vi "_USB_CAN_DISP_ID_HB_.vi"(1 "arr new":T1[](array[typedef]), 2 "Reset buffer":bool, 3 "arr old":T1[](array[typedef])) -> (0 "Arr Out":T1[](array[typedef]))   [LabVIEW 2011]
uses:
  _USB_CAN_T_R_Unit_.ctl
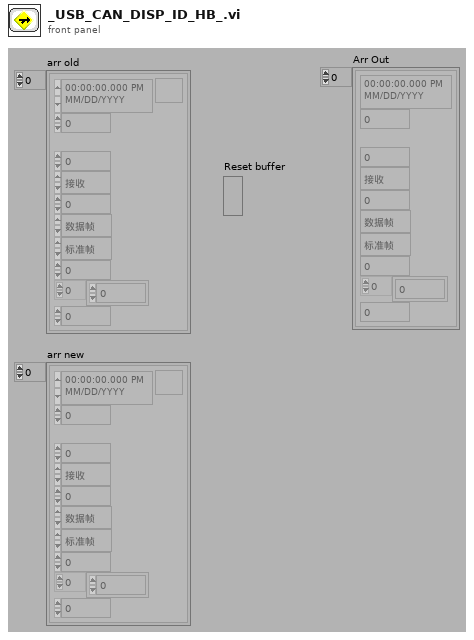
[diagram p1: front panel]
types:
  T1 = typedef "_USB_CAN_T_R_Unit_.ctl" = cluster{"time":timestamp, "channel":u16, "TimeStamp":u32, "tr":enum16{"接收", "发送"}, "id":u32, "Type":enum16{"数据帧", "远程帧"}, "Format":enum16{"标准帧", "扩展帧"}, "len":u8, "data":u8[], "sysTime":u32}
  T2 = cluster{"sysTime":u32, "channel":u16, "tr":enum16{"接收", "发送"}, "TR_Unit":T1}
  T3 = cluster{"sysTime":u32, "channel":u16, "tr":enum16{"接收", "发送"}, "TR_Unit":T1}[]
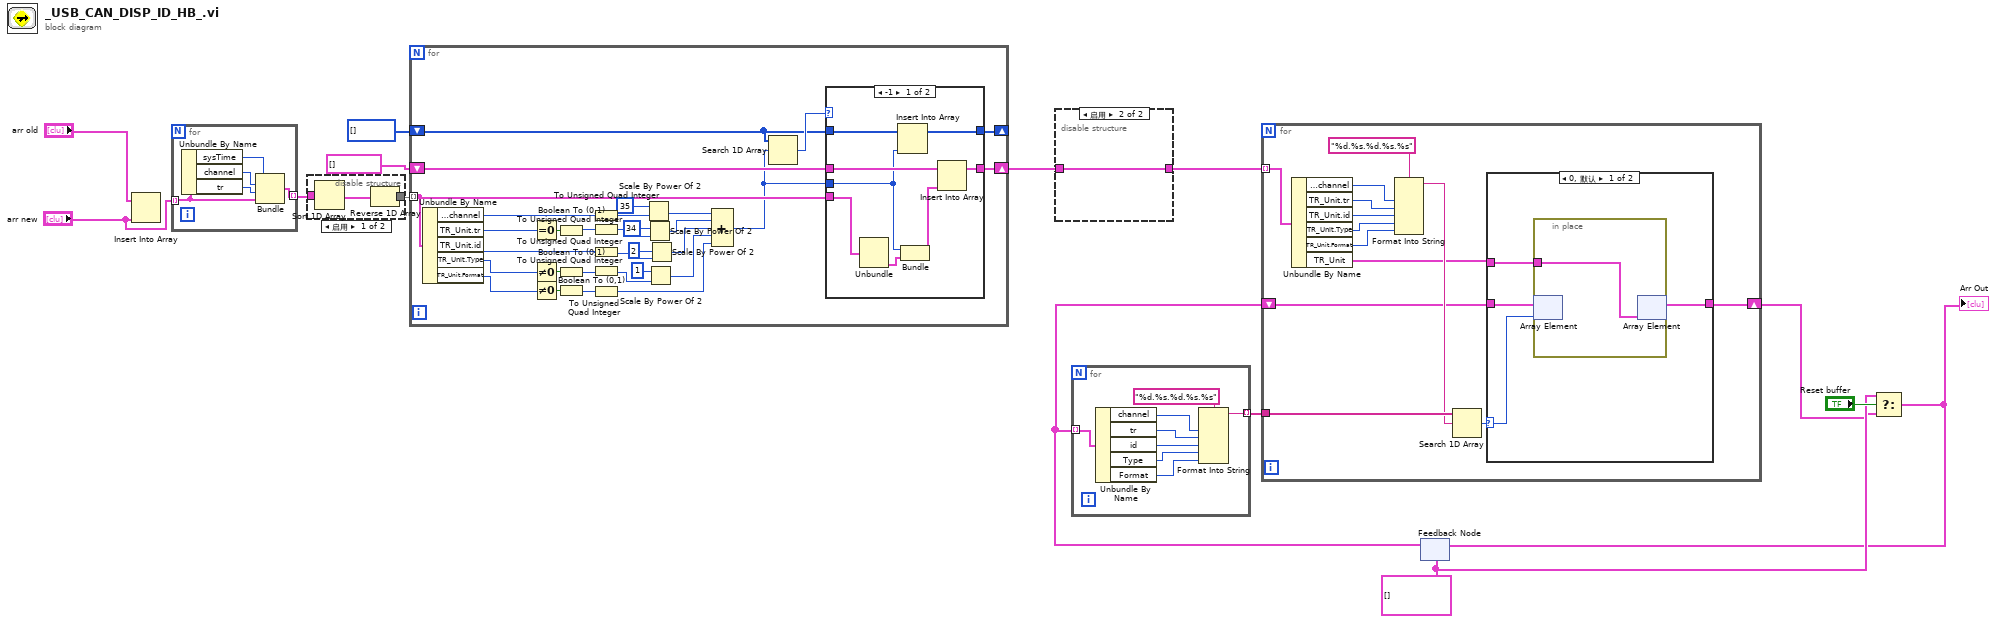
[diagram p0: block diagram]
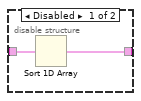
[diagram p2: hidden frame]
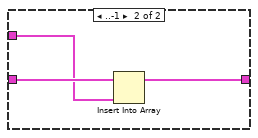
[diagram p4: hidden frame]
diagram:
  w4 = T1[] []
  n1 = Insert Into Array(array="arr old", new element="arr new") -> ()  [unwired: 1 in, 1 out]
  n2 = for {
    tunnel: "arr new" -> [w19] mode=indexing
    tunnel: [w17] -> w9 mode=indexing
    n3 = Unbundle By Name(w19) -> ("sysTime"=w15:u32, "channel"=w16:u16, "tr"=w18:enum16{"接收", "发送"})
    n4 = Bundle("sysTime"=w15, "channel"=w16, "tr"=w18, "TR_Unit"=w19) -> (w17:T2)  [unwired: 1 in]
  }
  n5 = disable-structure shown="启用" {
    disable-tunnel: w9 -> [w22 w23]
    disable-tunnel: [w20 w23] -> w8
    frame Enabled {
      n6 = Sort 1D Array(array=w22) -> (sorted array=w21:T3)
      n7 = Reverse 1D Array(array=w21) -> (reversed array=w20:T3)
    }
    frame Disabled {
    }
  }
  n8 = for {
    tunnel: w8 -> [w49] mode=indexing
    shift-right: [w52] -> w13
    shift-left: cluster{u64, "TR_Unit":T1}[] [] -> [w53]
    shift-right: [w50] -> _
    shift-left: u64[] [] -> [w51]
    n9 = Unbundle By Name(w49) -> ("TR_Unit.channel"=w28:u16, "TR_Unit.tr"=w27:enum16{"接收", "发送"}, "TR_Unit.id"=w24:u32, "TR_Unit.Type"=w26:enum16{"数据帧", "远程帧"}, "TR_Unit.Format"=w25:enum16{"标准帧", "扩展帧"})
    n10 = Equal To 0?(x=w27) -> (x = 0?=w48:bool)
    n11 = Not Equal To 0?(x=w26) -> (x != 0?=w47:bool)
    n12 = Not Equal To 0?(x=w25) -> (x != 0?=w46:bool)
    n13 = Boolean To (0,1)(Boolean=w48) -> (0, 1=w45:i16)
    n14 = Boolean To (0,1)(Boolean=w47) -> (0, 1=w44:i16)
    n15 = Boolean To (0,1)(Boolean=w46) -> (0, 1=w43:i16)
    n16 = To Unsigned Quad Integer(1:w28) -> (0:w42:u64)
    n17 = To Unsigned Quad Integer(1:w45) -> (0:w40:u64)
    n18 = To Unsigned Quad Integer(1:w24) -> (0:w38:u64)
    n19 = To Unsigned Quad Integer(1:w44) -> (0:w36:u64)
    n20 = To Unsigned Quad Integer(1:w43) -> (0:w30:u64)
    n21 = Scale By Power Of 2(n=35, x=w42) -> (x*2^n=w34:u64)
    n22 = Scale By Power Of 2(n=34, x=w40) -> (x*2^n=w33:u64)
    n23 = Scale By Power Of 2(n=1, x=w36) -> (x*2^n=w31:u64)
    n24 = Scale By Power Of 2(n=2, x=w38) -> (x*2^n=w32:u64)
    n25 = Compound Arithmetic op=ADD(w34, w33, w32, w31, w30) -> (w29:u64)
    n26 = Search 1D Array(1D array=w51, element=w29) -> (index of element=w54:i32)  [unwired: 1 in]
    n27 = case shown="-1" w54 {
      tunnel: w29 -> [w57 _]
      tunnel: w53 -> [w60 w63]
      tunnel: [w59 w63] -> w52
      tunnel: w51 -> [w62 w64]
      tunnel: [w61 w64] -> w50
      tunnel: w49 -> [w58 _]
      frame -1 {
        n28 = Unbundle(w58) -> ("TR_Unit"=w55:T1)  [unwired: 3 out]
        n29 = Insert Into Array(array=w62, new element=w57) -> (w61:u64[])  [unwired: 1 in]
        n30 = Bundle(w57, "TR_Unit"=w55) -> (w56:cluster{u64, "TR_Unit":T1})  [unwired: 1 in]
        n31 = Insert Into Array(array=w60, new element=w56) -> (w59:cluster{u64, "TR_Unit":T1}[])  [unwired: 1 in]
      }
      frame 0, Default {
      }
    }
  }
  n32 = disable-structure shown="启用" {
    disable-tunnel: w13 -> [w66 w67]
    disable-tunnel: [w65 w67] -> w12
    frame Disabled {
      n33 = Sort 1D Array(array=w66) -> (sorted array=w65:cluster{u64, "TR_Unit":T1}[])
    }
    frame Enabled {
    }
  }
  n34 = feedback #1(w4) -> (w6:T1[])
  n35 = for {
    tunnel: w6 -> [w75] mode=indexing
    tunnel: [w70] -> w7 mode=indexing
    n36 = Unbundle By Name(w75) -> ("channel"=w74:u16, "tr"=w73:enum16{"接收", "发送"}, "id"=w72:u32, "Type"=w69:enum16{"数据帧", "远程帧"}, "Format"=w68:enum16{"标准帧", "扩展帧"})
    n37 = Format Into String(format string="%d.%s.%d.%s.%s" ("格式字符串"), w74, w73, w72, w69, w68) -> (resulting string=w70:string)  [unwired: 2 in, 1 out]
  }
  n38 = for {
    tunnel: w12 -> [w76] mode=indexing
    tunnel: w7 -> [w84]
    shift-right: [w80] -> w3
    shift-left: w6 -> [w81]
    n39 = Unbundle By Name(w76) -> ("TR_Unit.channel"=w85:u16, "TR_Unit.tr"=w86:enum16{"接收", "发送"}, "TR_Unit.id"=w87:u32, "TR_Unit.Type"=w78:enum16{"数据帧", "远程帧"}, "TR_Unit.Format"=w77:enum16{"标准帧", "扩展帧"}, "TR_Unit"=w79:T1)
    n40 = Format Into String(format string="%d.%s.%d.%s.%s" ("格式字符串"), w85, w86, w87, w78, w77) -> (resulting string=w83:string)  [unwired: 2 in, 1 out]
    n41 = Search 1D Array(1D array=w84, element=w83) -> (index of element=w82:i32)  [unwired: 1 in]
    n42 = case shown="0, 默认" w82 {
      selector: w82 -> [w91 _]
      tunnel: w81 -> [w92 w96]
      tunnel: w79 -> [w90 w95]
      tunnel: [w89 w94] -> w80
      frame 0, Default {
        n43 = in-place {
          in-place-border: w90 -> [w93]
          n44 = in-place-array #2(w92, w91) -> ()  [unwired: 1 out]
          n45 = in-place-array #2(w93) -> (w89:T1[])  [unwired: 1 out]
        }
      }
      frame ..-1 {
        n46 = Insert Into Array(array=w96, new element=w95) -> (w94:T1[])  [unwired: 1 in]
      }
    }
  }
  n47 = Select(t=w4, s="Reset buffer", f=w3) -> (s? t:f=w2:T1[])
  "Arr Out" <- w2
  n48 = feedback-in #1(w2) -> ()
